vi "PurePursuitTester.vi"() -> ()   [LabVIEW 2016]
uses:
  <vilib>/Rock Robotics/WPI/Utilities/WPI_GetSetVariantRefNum.vi
panel:
  in  "Trackwidth":dbl=40.0 format="%#_13g"
  in  "Max Accel":dbl=65.0 format="%#_13g"
  in  "GO":bool
  in  "Average Vels":bool
  out "Output":cluster{"r":dbl, "dx/dt":dbl}(graph)={"r"=-0.04423077432905621, "dx/dt"=-0.03941356210525552}
  in  "Gains":T1={"FFV"=0.0088, "FFA"=0.0017, "Vel PID"={"P"=0.01, "I"=0.007, "D"=0.0}} {"Vel PID"."D" format="%.3f"; "Vel PID"."I" format="%.3f"; "Vel PID"."P" format="%.3f"}
  out "Vel Right":cluster{"r":dbl, "dx/dt":dbl}(graph)
  out "Vel Left":cluster{"l":dbl, "dx/dt":dbl}(graph)
  out "Graph":cluster{cluster{"x":dbl, "y":dbl}[]}[](graph)=[{[{"x"=0.0, "y"=0.0}, {"x"=6.123233995736766e-17, "y"=1.0}, {"x"=1.2246467991473532e-16, "y"=2.0}, {"x"=1.8369701987210297e-16, "y"=3.0}, {"x"=2.4492935982947064e-16, "y"=4.0}, {"x"=3.061616997868383e-16, "y"=5.0}, {"x"=3.6739403974420594e-16, "y"=6.0}, {"x"=4.286263797015736e-16, "y"=7.0}, {"x"=4.898587196589413e-16, "y"=8.0}, {"x"=5.51091059616309e-16, "y"=9.0}, {"x"=6.123233995736766e-16, "y"=10.0}, {"x"=6.735557395310443e-16, "y"=11.0}, {"x"=7.347880794884119e-16, "y"=12.0}, {"x"=7.960204194457795e-16, "y"=13.0}, {"x"=8.572527594031472e-16, "y"=14.0}, {"x"=9.18485099360515e-16, "y"=15.0}, {"x"=9.797174393178826e-16, "y"=16.0}, {"x"=1.0409497792752501e-15, "y"=17.0}, {"x"=1.102182119232618e-15, "y"=18.0}, {"x"=1.1634144591899855e-15, "y"=19.0}, {"x"=1.2246467991473533e-15, "y"=20.0}, {"x"=1.2858791391047208e-15, "y"=21.0}, {"x"=1.3471114790620886e-15, "y"=22.0}, {"x"=1.4083438190194562e-15, "y"=23.0}, {"x"=1.4695761589768238e-15, "y"=24.0}, {"x"=1.5308084989341915e-15, "y"=25.0}, {"x"=1.592040838891559e-15, "y"=26.0}, {"x"=1.6532731788489269e-15, "y"=27.0}, {"x"=1.7145055188062944e-15, "y"=28.0}, {"x"=1.7757378587636622e-15, "y"=29.0}, {"x"=1.83697019872103e-15, "y"=30.0}, {"x"=1.8982025386783976e-15, "y"=31.0}, {"x"=1.959434878635765e-15, "y"=32.0}, {"x"=2.0206672185931327e-15, "y"=33.0}, {"x"=2.0818995585505003e-15, "y"=34.0}, {"x"=2.1431318985078682e-15, "y"=35.0}, {"x"=2.204364238465236e-15, "y"=36.0}, {"x"=2.2655965784226034e-15, "y"=37.0}, {"x"=2.326828918379971e-15, "y"=38.0}, {"x"=2.388061258337339e-15, "y"=39.0}, {"x"=2.4492935982947065e-15, "y"=40.0}, {"x"=2.510525938252074e-15, "y"=41.0}, {"x"=2.5717582782094417e-15, "y"=42.0}, {"x"=2.6329906181668092e-15, "y"=43.0}, {"x"=2.6942229581241772e-15, "y"=44.0}, {"x"=2.7554552980815448e-15, "y"=45.0}, {"x"=0.0, "y"=46.0}, {"x"=0.8320502943378437, "y"=46.55470019622523}, {"x"=1.6641005886756874, "y"=47.10940039245046}, {"x"=2.4961508830135313, "y"=47.66410058867569}, {"x"=3.328201177351375, "y"=48.218800784900914}, {"x"=4.160251471689219, "y"=48.77350098112615}, {"x"=4.9923017660270625, "y"=49.328201177351374}, {"x"=5.824352060364906, "y"=49.8829013735766}, {"x"=6.65640235470275, "y"=50.437601569801835}, {"x"=7.488452649040593, "y"=50.99230176602706}, {"x"=8.320502943378438, "y"=51.54700196225229}, {"x"=9.152553237716281, "y"=52.10170215847752}, {"x"=9.984603532054125, "y"=52.65640235470275}, {"x"=10.816653826391969, "y"=53.211102550927976}, {"x"=11.648704120729812, "y"=53.76580274715321}, {"x"=12.480754415067656, "y"=54.320502943378436}, {"x"=13.3128047094055, "y"=54.87520313960366}, {"x"=14.144855003743343, "y"=55.4299033358289}, {"x"=14.976905298081187, "y"=55.98460353205412}, {"x"=15.80895559241903, "y"=56.53930372827935}, {"x"=16.641005886756876, "y"=57.09400392450458}, {"x"=17.47305618109472, "y"=57.64870412072981}, {"x"=18.305106475432563, "y"=58.20340431695504}, {"x"=19.137156769770407, "y"=58.75810451318027}, {"x"=19.96920706410825, "y"=59.3128047094055}, {"x"=20.801257358446094, "y"=59.867504905630724}, {"x"=21.633307652783937, "y"=60.42220510185595}, {"x"=22.46535794712178, "y"=60.976905298081185}, {"x"=23.297408241459625, "y"=61.53160549430641}, {"x"=24.12945853579747, "y"=62.086305690531645}, {"x"=24.961508830135312, "y"=62.64100588675687}, {"x"=25.793559124473155, "y"=63.1957060829821}, {"x"=26.625609418811, "y"=63.750406279207326}, {"x"=27.457659713148843, "y"=64.30510647543255}, {"x"=28.289710007486686, "y"=64.8598066716578}, {"x"=29.12176030182453, "y"=65.41450686788302}, {"x"=29.953810596162374, "y"=65.96920706410825}, {"x"=30.785860890500217, "y"=66.52390726033347}, {"x"=31.61791118483806, "y"=67.0786074565587}, {"x"=32.449961479175904, "y"=67.63330765278394}, {"x"=33.28201177351375, "y"=68.18800784900915}, {"x"=34.11406206785159, "y"=68.7427080452344}, {"x"=34.94611236218944, "y"=69.29740824145962}, {"x"=35.77816265652728, "y"=69.85210843768485}, {"x"=36.610212950865126, "y"=70.40680863391007}, {"x"=37.442263245202966, "y"=70.9615088301353}, {"x"=38.27431353954081, "y"=71.51620902636054}, {"x"=39.10636383387865, "y"=72.07090922258577}, {"x"=39.9384141282165, "y"=72.625609418811}, {"x"=40.77046442255434, "y"=73.18030961503622}, {"x"=41.60251471689219, "y"=73.73500981126145}, {"x"=42.43456501123003, "y"=74.28971000748668}, {"x"=43.266615305567875, "y"=74.8444102037119}, {"x"=44.098665599905715, "y"=75.39911039993714}, {"x"=44.93071589424356, "y"=75.95381059616237}, {"x"=45.7627661885814, "y"=76.5085107923876}, {"x"=46.59481648291925, "y"=77.06321098861282}, {"x"=47.42686677725709, "y"=77.61791118483805}, {"x"=48.25891707159494, "y"=78.17261138106329}, {"x"=49.09096736593278, "y"=78.7273115772885}, {"x"=49.923017660270624, "y"=79.28201177351374}, {"x"=50.755067954608464, "y"=79.83671196973897}, {"x"=51.58711824894631, "y"=80.3914121659642}, {"x"=52.41916854328415, "y"=80.94611236218944}, {"x"=53.251218837622, "y"=81.50081255841465}, {"x"=54.083269131959845, "y"=82.05551275463989}, {"x"=54.915319426297685, "y"=82.61021295086512}, {"x"=55.74736972063553, "y"=83.16491314709035}, {"x"=56.57942001497337, "y"=83.71961334331557}, {"x"=57.41147030931122, "y"=84.2743135395408}, {"x"=58.24352060364906, "y"=84.82901373576604}, {"x"=59.07557089798691, "y"=85.38371393199125}, {"x"=59.90762119232475, "y"=85.9384141282165}, {"x"=60.739671486662594, "y"=86.49311432444172}, {"x"=61.571721781000434, "y"=87.04781452066695}, {"x"=62.40377207533828, "y"=87.60251471689219}, {"x"=63.23582236967612, "y"=88.1572149131174}, {"x"=64.06787266401396, "y"=88.71191510934264}, {"x"=64.89992295835181, "y"=89.26661530556787}, {"x"=65.73197325268966, "y"=89.8213155017931}, {"x"=66.5640235470275, "y"=90.37601569801832}, {"x"=67.39607384136534, "y"=90.93071589424355}, {"x"=68.22812413570318, "y"=91.48541609046879}, {"x"=69.06017443004103, "y"=92.040116286694}, {"x"=69.89222472437888, "y"=92.59481648291924}, {"x"=70.72427501871671, "y"=93.14951667914447}, {"x"=71.55632531305456, "y"=93.7042168753697}, {"x"=72.3883756073924, "y"=94.25891707159494}, {"x"=73.22042590173025, "y"=94.81361726782015}, {"x"=74.05247619606808, "y"=95.36831746404539}, {"x"=74.88452649040593, "y"=95.92301766027062}, {"x"=75.71657678474378, "y"=96.47771785649584}, {"x"=76.54862707908163, "y"=97.03241805272107}, {"x"=77.25, "y"=97.5}]}, {[{"x"=78.74238592743468, "y"=99.11996794477173}, {"x"=88.76056028659556, "y"=105.72573682579167}]}, {[{"x"=77.25, "y"=97.5}]}, {[{"x"=108.74238592743468, "y"=99.11996794477173}, {"x"=107.27408141628929, "y"=108.39047777602015}, {"x"=103.0128957586831, "y"=116.75352551354592}, {"x"=96.37594349620888, "y"=123.39047777602016}, {"x"=88.0128957586831, "y"=127.65166343362634}, {"x"=78.74238592743468, "y"=129.11996794477173}, {"x"=69.47187609618626, "y"=127.65166343362634}, {"x"=61.10882835866049, "y"=123.39047777602016}, {"x"=54.471876096186264, "y"=116.75352551354592}, {"x"=50.21069043858007, "y"=108.39047777602016}, {"x"=48.74238592743468, "y"=99.11996794477173}, {"x"=50.21069043858007, "y"=89.84945811352331}, {"x"=54.47187609618626, "y"=81.48641037599754}, {"x"=61.10882835866049, "y"=74.84945811352331}, {"x"=69.47187609618625, "y"=70.58827245591712}, {"x"=78.74238592743468, "y"=69.11996794477173}, {"x"=88.0128957586831, "y"=70.58827245591712}, {"x"=96.37594349620886, "y"=74.8494581135233}, {"x"=103.0128957586831, "y"=81.48641037599754}, {"x"=107.27408141628929, "y"=89.8494581135233}, {"x"=108.74238592743468, "y"=99.11996794477172}]}, {[{"x"=1392.9638722644045, "y"=-608.515394016017}, {"x"=1351.4783018615326, "y"=-346.5858110477284}, {"x"=1231.0824873309166, "y"=-110.29572063109106}, {"x"=1043.5616098457772, "y"=77.22515685404824}, {"x"=807.2715194291399, "y"=197.62097138466447}, {"x"=545.3419364608512, "y"=239.10654178753612}, {"x"=283.41235349256266, "y"=197.62097138466459}, {"x"=47.12226307592539, "y"=77.22515685404824}, {"x"=-140.3986144092139, "y"=-110.295720631091}, {"x"=-260.79442893983025, "y"=-346.5858110477283}, {"x"=-302.2799993427019, "y"=-608.5153940160169}, {"x"=-260.79442893983037, "y"=-870.4449769843055}, {"x"=-140.39861440921402, "y"=-1106.7350674009429}, {"x"=47.12226307592522, "y"=-1294.255944886082}, {"x"=283.4123534925625, "y"=-1414.6517594166985}, {"x"=545.3419364608511, "y"=-1456.1373298195701}, {"x"=807.2715194291397, "y"=-1414.6517594166985}, {"x"=1043.561609845777, "y"=-1294.2559448860823}, {"x"=1231.0824873309164, "y"=-1106.735067400943}, {"x"=1351.4783018615326, "y"=-870.4449769843059}, {"x"=1392.9638722644045, "y"=-608.5153940160172}]}]
  in  "Vel":dbl=85.0
  in  "LookAhead":dbl(slide)=30.0 scale=0.0..50.0
  in  "Path":cluster{"x":dbl, "y":dbl}[](array[cluster])=[{"x"=0.0, "y"=0.0}, {"x"=0.0, "y"=46.0}, {"x"=77.25, "y"=97.5}]
  # "SET DEFAULTS"
  # "72"
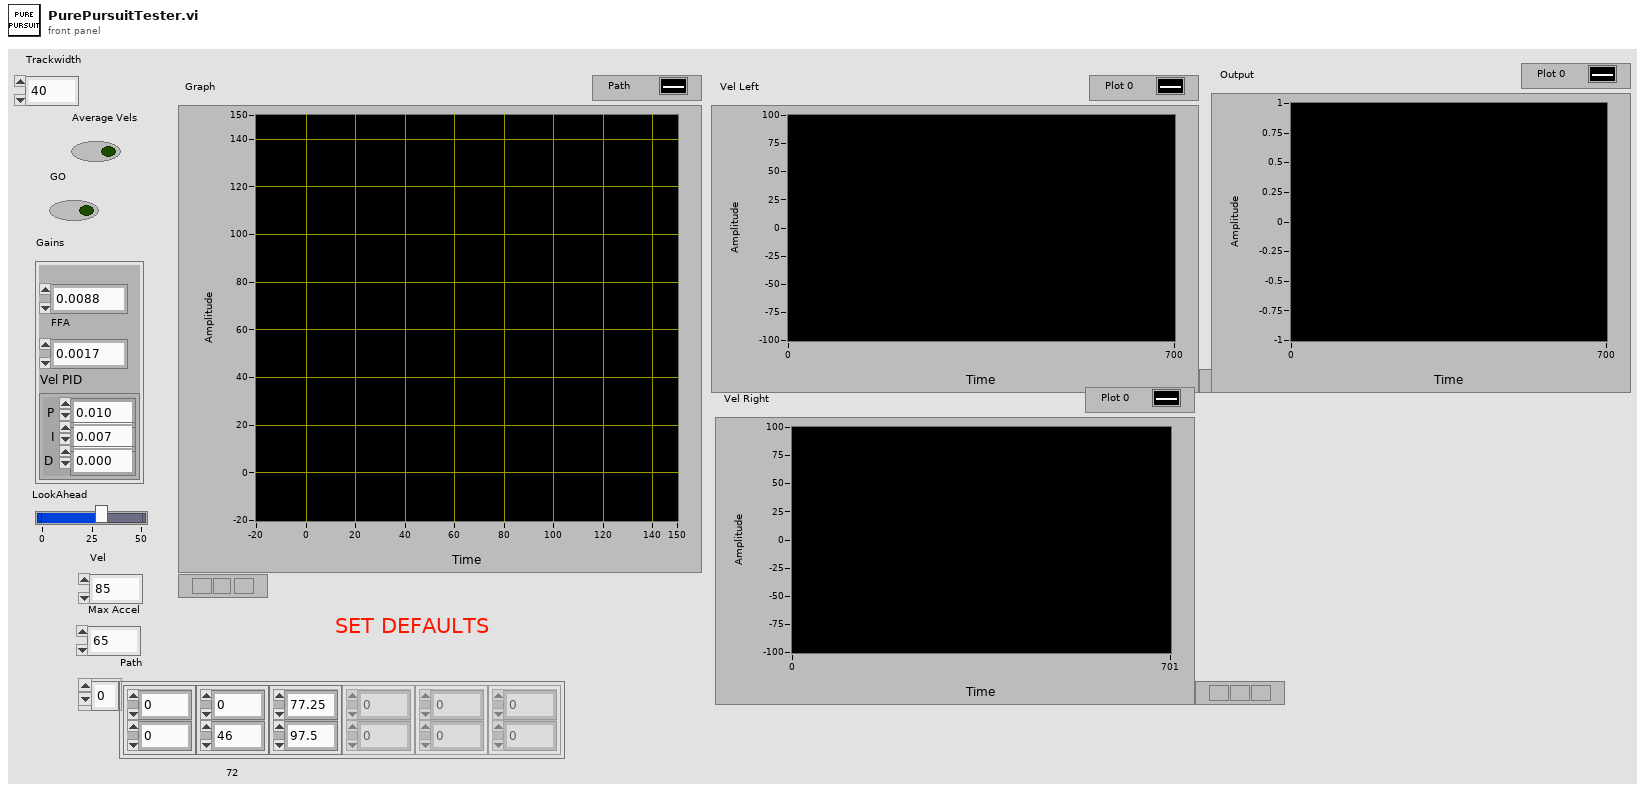
[diagram p1: front panel]
types:
  T1 = cluster{"FFV":dbl, "FFA":dbl, "Vel PID":cluster{"P":dbl, "I":dbl, "D":dbl}}
  T2 = typedef "WPI_EncoderDevRef.ctl" = cluster{"DevStatus":errorcluster, "EncoderIndex":T3, "CounterIndex":T4, "DistancePerCount":dbl, "Decoding Type":T5}
  T3 = typedef "FPGA_EncoderIdx.ctl" = enum8{"Enc 0", "Enc 1", "Enc 2", "Enc 3", "Enc 4", "Enc 5", "Enc 6", "Enc 7", "Invalid"}
  T4 = typedef "FPGA_CounterCtrSystemIndex.ctl" = enum8{"Ctr 0", "Ctr 1", "Ctr 2", "Ctr 3", "Ctr 4", "Ctr 5", "Ctr 6", "Ctr 7", "Invalid"}
  T5 = typedef "WPI_EncoderType.ctl" = enum16{"1x", "2x", "4x"}
  T6 = typedef "WPI_RobotDriveDevRef.ctl" = cluster{"DevStatus":errorcluster, "Motors[]":T7[], "Square Inputs":bool, "Max Output":dbl}
  T7 = typedef "WPI_MotorControlDeviceRef.ctl" = cluster{"DeviceStatus":errorcluster, "Type":T8, "PWM":cluster{"PWM Channel":T9, "DeadBand":T10}, "CAN":cluster{"Device Number":u8, "SetOutput VI Ref":variant, "GetOutput VI Ref":variant, "Enable VI Ref":variant, "Disable VI Ref":variant, "Data":variant}, "Invert":bool}
  T8 = typedef "WPI_MotorControlType.ctl" = enum16{"PWM", "CAN"}
  T9 = typedef "FPGA_DIOPWMChannel.ctl" = enum8{"PWM 0", "PWM 1", "PWM 2", "PWM 3", "PWM 4", "PWM 5", "PWM 6", "PWM 7", "PWM 8", "PWM 9", "PWM MXP 0", "PWM MXP 1", "PWM MXP 2", "PWM MXP 3", "PWM MXP 4", "PWM MXP 5", "PWM MXP 6", "PWM MXP 7", "PWM MXP 8", "PWM MXP 9", "Invalid"}
  T10 = typedef "WPI_PWMDeadband.ctl" = cluster{"Name":string, "maxPositivePwm":i32, "minPositivePwm":i32, "centerPwm":i32, "maxNegativePwm":i32, "minNegativePwm":i32, "angularRange":u16}
  T11 = cluster{"Yaw":dbl, "Roll":dbl, "Pitch":dbl, "Heading":dbl, "Fused Heading":dbl}
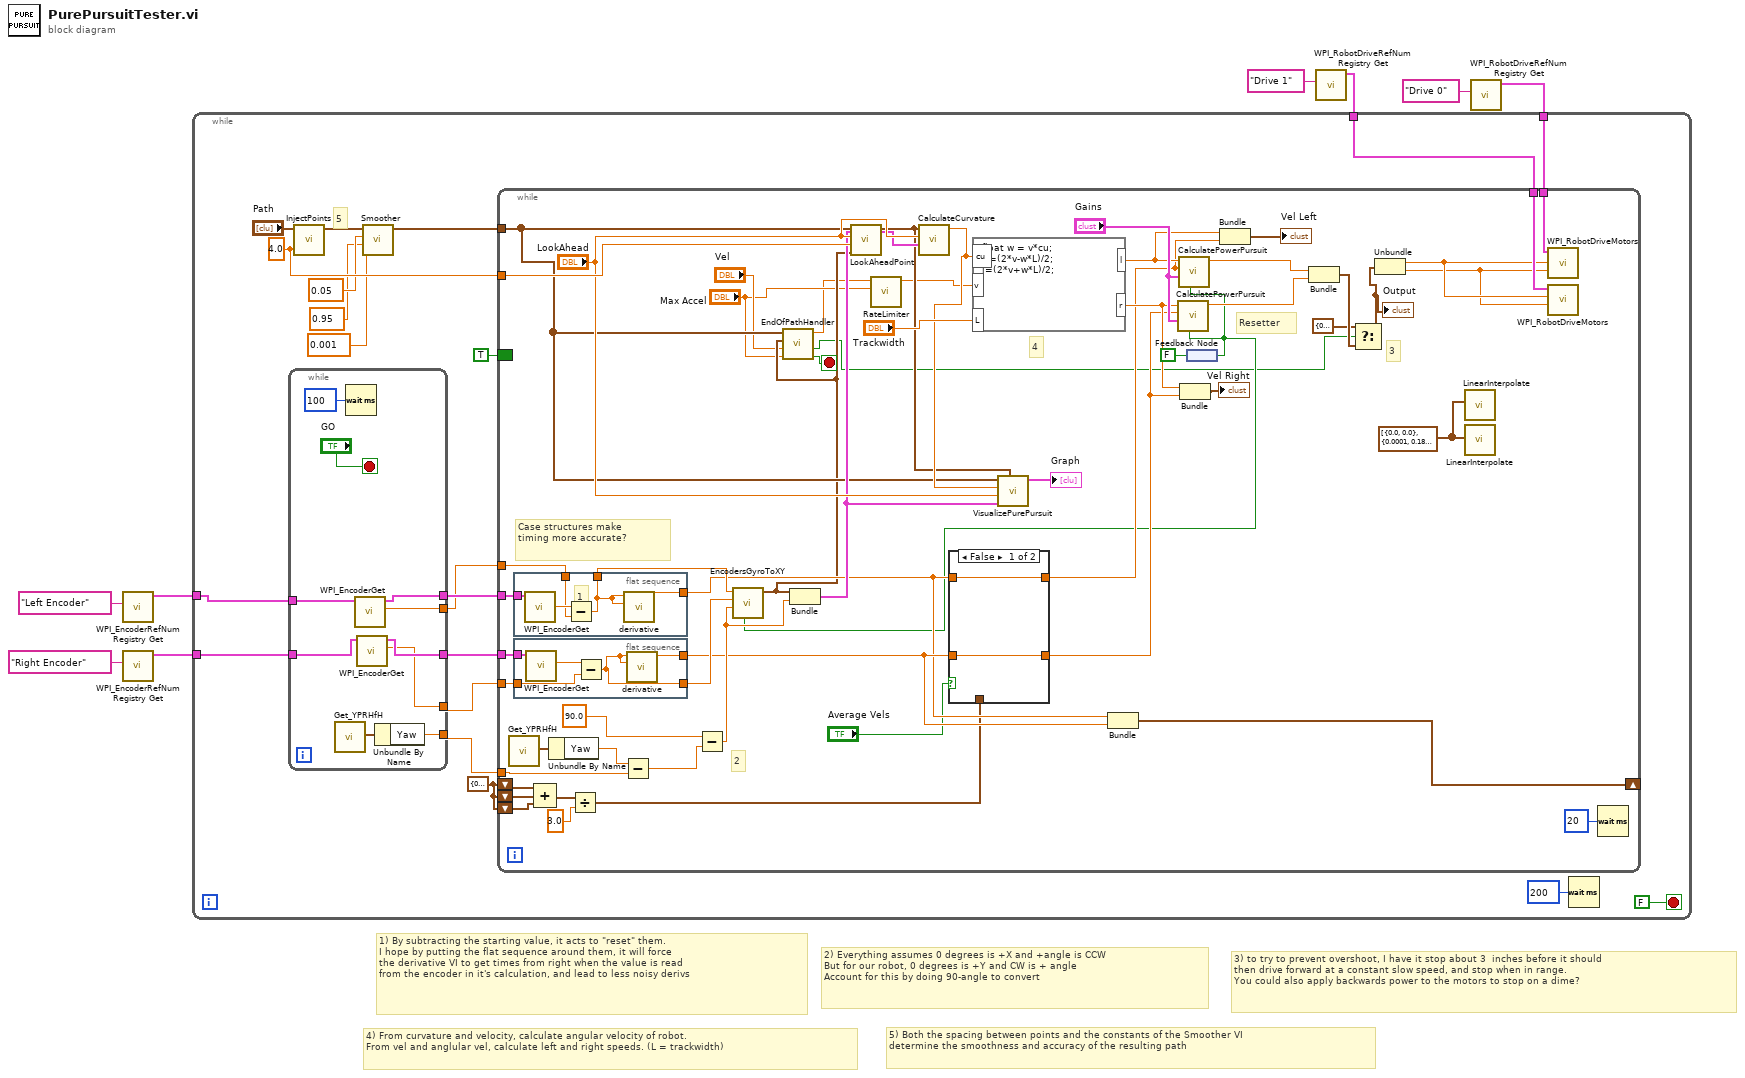
[diagram p0: block diagram]
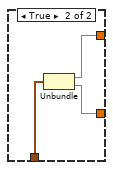
[diagram p2: hidden frame]
diagram:
  # "5) Both the spacing between points and the constants of the Smoother VI\ndetermine the smoothness and accuracy of the resulting path"
  # "4) From curvature and velocity, calculate angular velocity of robot.\nFrom vel and anglular vel, calculate left and right speeds. (L = trackwidth)"
  # "3) to try to prevent overshoot, I have it stop about 3  inches before it should\nthen drive forward at a constant slow speed, and stop when in range. \nYou could also apply backwards power to the motors to stop on a dime?"
  # "2) Everything assumes 0 degrees is +X and +angle is CCW\nBut for our robot, 0 degrees is +Y and CW is + angle\nAccount for this by doing 90-angle to convert"
  # "1) By subtracting the starting value, it acts to \"reset\" them.\nI hope by putting the flat sequence around them, it will force\nthe derivative VI to get times from right when the value is read\nfrom the encoder in it's calculation, and lead to less noisy derivs"
  n1 = call <vilib>:"WPI_EncoderRefNum Registry Get.vi"("refnum name"="Left Encoder") -> ("EncoderDevRef"=w4:T2)  [unwired: 9 in, 1 out]
  n2 = call <vilib>:"WPI_EncoderRefNum Registry Get.vi"("refnum name"="Right Encoder") -> ("EncoderDevRef"=w3:T2)  [unwired: 9 in, 1 out]
  n3 = call <vilib>:"WPI_RobotDriveRefNum Registry Get.vi"("refnum name"="Drive 1") -> ("RobotDriveDevRef"=w1:T6)  [unwired: 9 in, 1 out]
  n4 = call <vilib>:"WPI_RobotDriveRefNum Registry Get.vi"("refnum name"="Drive 0") -> ("RobotDriveDevRef"=w7:T6)  [unwired: 9 in, 1 out]
  n5 = while {
    tunnel: w7 -> [w26]
    tunnel: w4 -> [w19]
    tunnel: w3 -> [w17]
    tunnel: w1 -> [w21]
    stop <- FALSE stop-if-true
    w25 = cluster{"dx/dt":dbl, "dx/dt":dbl} {"dx/dt"=0.0, "dx/dt"=0.0}
    w27 = 4.0 ("Distance")
    # "5"
    n6 = while {
      tunnel: [w35] -> w20
      tunnel: w19 -> [w34]
      tunnel: [w33] -> w18
      tunnel: w17 -> [w32]
      tunnel: [w31] -> w16
      tunnel: [w30] -> w15
      tunnel: [w29] -> w14
      stop <- "GO" stop-if-true
      n7 = call <vilib>:"Get_YPRHfH.vi"() -> ("YRPHfH"=w36:T11)  [unwired: 11 in]
      n8 = Wait (ms)(milliseconds to wait=u32 100) -> ()  [unwired: 1 out]
      n9 = call <vilib>:"WPI_EncoderGet.vi"("EncoderDevRef"=w34) -> ("Distance"=w29:dbl, "EncoderDevRef"=w33:T2)  [unwired: 5 in, 4 out]
      n10 = call <vilib>:"WPI_EncoderGet.vi"("EncoderDevRef"=w32) -> ("Distance"=w30:dbl, "EncoderDevRef"=w31:T2)  [unwired: 5 in, 4 out]
      n11 = Unbundle By Name(w36) -> ("Yaw"=w35:dbl)
    }
    n12 = call "InjectPoints.vi"("Distance"=w27, "Path"="Path") -> ("Path out"=w13:cluster{dbl, dbl}[])  [unwired: 9 in]
    n13 = call "Smoother.vi"("tolerance"=0.001, "B"=0.95, "A"=0.05, "Path"=w13) -> ("Smooth Path"=w12:cluster{"x":dbl, "y":dbl}[])  [unwired: 7 in]
    n14 = while {
      tunnel: w12 -> [w56]
      tunnel: w18 -> [w94]
      tunnel: w16 -> [w93]
      tunnel: w27 -> [w90]
      tunnel: w26 -> [w82]
      tunnel: w21 -> [w81]
      shift-right: [w73] -> _
      shift-left: w25 -> [w72]
      shift-left: w25 -> [w71]
      shift-left: w25 -> [w70]
      border: TRUE ("ENABLE") -> [_]
      tunnel: w20 -> [w49]
      tunnel: w15 -> [w47]
      tunnel: w14 -> [w46]
      stop <- w52 stop-if-true
      w43 = cluster{"X":dbl, "Y":dbl}[] [{"X"=0.0, "Y"=0.0}, {"X"=0.0001, "Y"=0.185}, {"X"=1.0, "Y"=1.0}] ("Points")
      # "4"
      # "3"
      # "2"
      # "Resetter"
      # "Case structures make\ntiming more accurate?"
      n15 = call <vilib>:"Get_YPRHfH.vi"() -> ("YRPHfH"=w92:T11)  [unwired: 11 in]
      n16 = flat-sequence {
        tunnel: w94 -> [w105]
        tunnel: [w104] -> w65
        tunnel: [w103] -> w86
        tunnel: w46 -> [w101]
        frame #0 {
          # "1"
          n17 = call <vilib>:"WPI_EncoderGet.vi"("EncoderDevRef"=w105) -> ("Distance"=w102:dbl)  [unwired: 5 in, 5 out]
          n18 = Subtract(x=w102, y=w101) -> (x-y=w103:dbl)
          n19 = call "derivative.vi"("Starting value"=w103, "x"=w103) -> ("dx/dt"=w104:dbl)  [unwired: 9 in]
        }
      }
      n20 = flat-sequence {
        tunnel: w93 -> [w110]
        tunnel: [w109] -> w67
        tunnel: [w107] -> w91
        tunnel: w47 -> [w106]
        frame #0 {
          n21 = call <vilib>:"WPI_EncoderGet.vi"("EncoderDevRef"=w110) -> ("Distance"=w108:dbl)  [unwired: 5 in, 5 out]
          n22 = Subtract(x=w108, y=w106) -> (x-y=w107:dbl)
          n23 = call "derivative.vi"("Starting value"=w107, "x"=w107) -> ("dx/dt"=w109:dbl)  [unwired: 9 in]
        }
      }
      n24 = Compound Arithmetic op=ADD(w72, w71, w70) -> (w69:cluster{"dx/dt":dbl, "dx/dt":dbl})
      n25 = Unbundle By Name(w92) -> ("Yaw"=w50:dbl)
      n26 = Divide(x=w69, y=3.0 ("x")) -> (x/y=w62:cluster{"dx/dt":dbl, "dx/dt":dbl})
      n27 = Subtract(x=w50, y=w49) -> (x-y=w48:dbl)
      n28 = Subtract(x=90.0, y=w48) -> (x-y=w79:dbl)
      n29 = case shown="False" "Average Vels" {
        tunnel: w67 -> [w97 _]
        tunnel: [w97 w99] -> w66
        tunnel: w65 -> [w96 _]
        tunnel: [w96 w100] -> w64
        tunnel: w62 -> [_ w98]
        frame False {
        }
        frame True {
          n30 = Unbundle(w98) -> ("dx/dt"=w100:dbl, "dx/dt"=w99:dbl)
        }
      }
      n31 = Bundle("dx/dt"=w65, "dx/dt"=w67) -> (w73:cluster{"dx/dt":dbl, "dx/dt":dbl})  [unwired: 1 in]
      n32 = feedback-in #1(FALSE ("ENABLE")) -> ()
      n33 = feedback #1() -> (w57:bool)
      n34 = call "EncodersGyroToXY.vi"("Reset"=w57, "Angle (degrees)"=w79, "Right Distance"=w91, "Left Distance"=w86) -> ("Location"=w55:cluster{dbl, dbl})  [unwired: 6 in, 1 out]
      n35 = call "EndOfPathHandler.vi"("MaxAccel"="Max Accel", "MaxVel"="Vel", "RobotLocation"=w55, "Path"=w56) -> ("Done"=w52:bool, "Override"=w41:bool, "VelOut"=w51:dbl)  [unwired: 4 in, 1 out]
      n36 = Bundle("Location"=w55, w79) -> (w75:cluster{"Location":cluster{dbl, dbl}, dbl})  [unwired: 1 in]
      n37 = call "LookAheadPoint.vi"("Robot"=w55, "Spacing"=w90, "LookAhead"="LookAhead", "Path"=w56) -> ("Point"=w74:cluster{"x":dbl, "y":dbl})  [unwired: 7 in]
      n38 = call "RateLimiter.vi"("Max dx/dt"="Max Accel", "Input"=w51) -> ("Output"=w59:dbl)  [unwired: 9 in]
      n39 = call "CalculateCurvature.vi"("Robot"=w75, "Lookahead"="LookAhead", "Point"=w74) -> ("Curvature"=w77:dbl)  [unwired: 8 in]
      n40 = formula code="float w = v*cu;\nr =(2*v-w*L)/2;\nl=(2*v+w*L)/2;"("L"="Trackwidth", "cu"=w77, "v"=w59) -> ("r"=w84:dbl, "l"=w87:dbl)
      n41 = call "VisualizePurePursuit.vi"("Lookahead Point"=w74, "Robot"=w75, "Lookahead"="LookAhead", "Curvature"=w77, "Path"=w56) -> ("Graph"=→"Graph":cluster{cluster{"x":dbl, "y":dbl}[]}[])  [unwired: 6 in]
      n42 = call "CalculatePowerPursuit.vi"("Reset"=w57, "Gains"="Gains", "Vel"=w66, "Target Vel"=w84) -> ("Power"=w60:dbl)  [unwired: 7 in]
      n43 = call "CalculatePowerPursuit.vi"("Reset"=w57, "Gains"="Gains", "Vel"=w64, "Target Vel"=w87) -> ("Power"=w61:dbl)  [unwired: 7 in]
      n44 = Bundle("r"=w84, "dx/dt"=w66) -> (→"Vel Right":cluster{"r":dbl, "dx/dt":dbl})  [unwired: 1 in]
      n45 = Bundle("l"=w87, "dx/dt"=w64) -> (→"Vel Left":cluster{"l":dbl, "dx/dt":dbl})  [unwired: 1 in]
      n46 = Bundle("Power"=w61, "Power"=w60) -> (w42:cluster{"Power":dbl, "Power":dbl})  [unwired: 1 in]
      n47 = Select(t=cluster{"Power":dbl, "Power":dbl} {"Power"=0.22, "Power"=0.22}, s=w41, f=w42) -> (s? t:f=w39:cluster{"Power":dbl, "Power":dbl})
      "Output" <- w39
      n48 = Unbundle(w39) -> ("Power"=w45:dbl, "Power"=w44:dbl)
      n49 = call "LinearInterpolate.vi"("Points"=w43) -> ()  [unwired: 10 in, 1 out]
      n50 = call "LinearInterpolate.vi"("Points"=w43) -> ()  [unwired: 10 in, 1 out]
      n51 = call <vilib>:"WPI_RobotDriveMotors.vi"("RightSpeed"=w44, "LeftSpeed"=w45, "RobotDriveDevRef"=w82) -> ()  [unwired: 6 in, 3 out]
      n52 = call <vilib>:"WPI_RobotDriveMotors.vi"("RightSpeed"=w44, "LeftSpeed"=w45, "RobotDriveDevRef"=w81) -> ()  [unwired: 6 in, 3 out]
      n53 = Wait (ms)(milliseconds to wait=u32 20) -> ()  [unwired: 1 out]
    }
    n54 = Wait (ms)(milliseconds to wait=u32 200) -> ()  [unwired: 1 out]
  }
